vi "mbtestmain.vi"() -> ()   [LabVIEW 2013, in "Modbus Slave tests.lvlib"]
doc: "Platypus Framework 1.0.1.65\nNI Systems Engineering - National Instruments"
uses:
  Modbus Slave tests.lvlib
  <vilib>/NI/Module Execution Interface/Engine Runtime/Engine Runtime Interface.lvclass
  <vilib>/NI/Module Execution Interface/Engine Runtime/Execution States.ctl
  execution/Modbus Slave runtime.lvclass
  <vilib>/NI/TBM Engines/Standard Engine/Runtime/Standard Engine Runtime.lvclass
  <vilib>/NI/TBM Modules/CVT Access/module/execution/CVT runtime.lvclass
  <vilib>/NI/Current Value Table/Current Value Table.lvlib
  <vilib>/NI/Current Value Table/DataTypes/Double_Read.vi
  <vilib>/NI/Current Value Table/DataTypes/Double_Write.vi
  <vilib>/NI/Current Value Table/DataTypes/Boolean_Read.vi
  <vilib>/NI/Current Value Table/DataTypes/Boolean_Write.vi
panel:
  in  "D":bool
  out "C":bool
  in  "B":dbl
  out "A":dbl
  in  "stop 2":bool
  out "final error":errorcluster
  in  "stop":bool
  out "runtime error":errorcluster
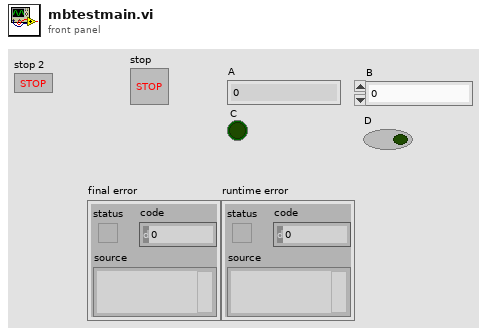
[diagram p1: front panel]
types:
  T1 = typedef "PLConfigurationSerializer.lvlib/systems cluster.ctl" = cluster{"System Configuration":refnum<class "PL_System Configuration.lvclass">, "targets":T2[]}
  T2 = typedef "PLConfigurationSerializer.lvlib/targets cluster.ctl" = cluster{"Target Configuration":refnum<class "PL_Target Configuration.lvclass">, "engines":T3[]}
  T3 = typedef "PLConfigurationSerializer.lvlib/engines cluster.ctl" = cluster{"engine configuration":refnum<class "engine configuration.lvclass">, "modules":refnum<class "TBM module configuration.lvclass">[]}
  T4 = typedef "Engine Runtime Interface.lvclass/Execution States.ctl" = enum16{"Initializing", "Paused (Initialized)", "Running", "Set Safe Outputs", "Uninitializing", "Stopped (Uninitialized)", "Error (Uninitialized)", "Safe State (Uninitialized)", "Closed"}
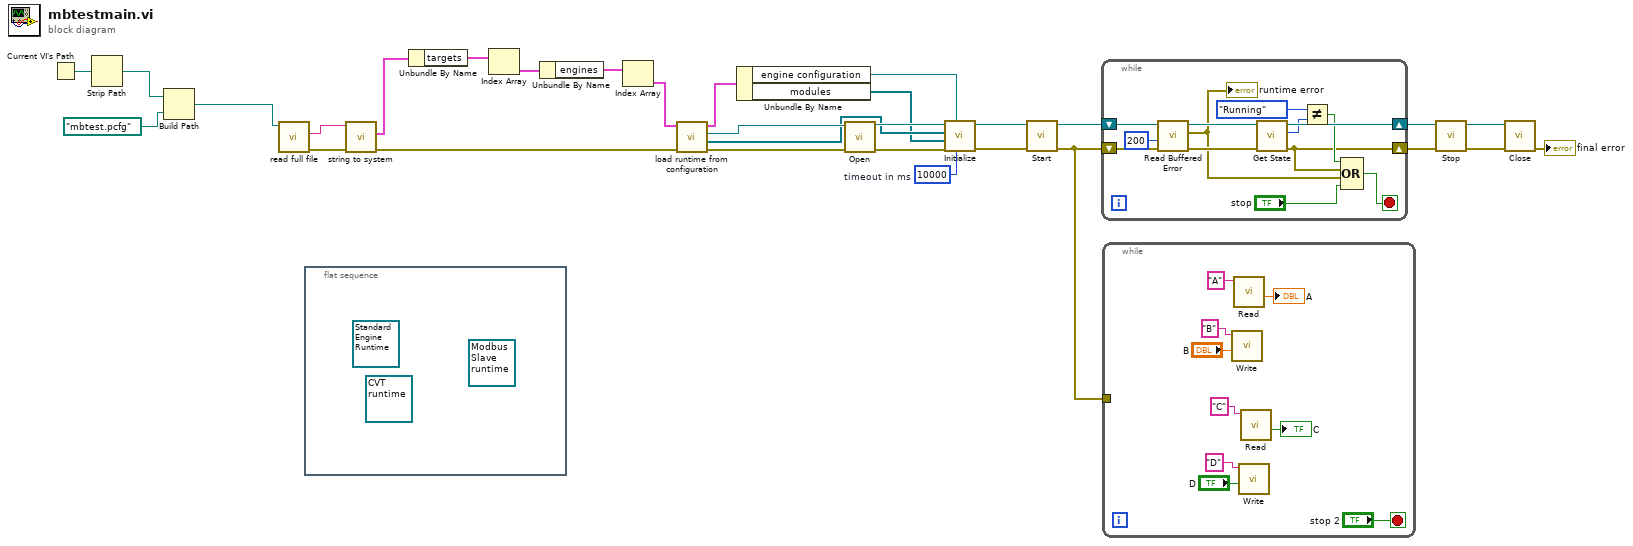
[diagram p0: block diagram]
diagram:
  w16 = 10000  # timeout in ms
  n1 = Current VI's Path() -> (path=w3:path)
  n2 = Strip Path(path=w3) -> (stripped path=w1:path)  [unwired: 1 out]
  n3 = Build Path(base path=w1, name or relative path=path "mbtest.pcfg" ("file path")) -> (appended path=w2:path)
  n4 = call <vilib>:"read full file.vi"("file path"=w2) -> ("error out"=w30:errorcluster, "data"=w29:string)  [unwired: 9 in]
  n5 = flat-sequence {
    frame #0 {
      (unwired) refnum<class "CVT runtime.lvclass"> refnum ("CVT runtime")
      (unwired) refnum<class "Standard Engine Runtime.lvclass"> refnum ("Standard Engine Runtime.lvclass")
      (unwired) refnum<class "Modbus Slave runtime.lvclass"> refnum ("Modbus Slave runtime")
    }
  }
  n6 = call <vilib>:"string to system.vi"("error in"=w30, "data"=w29) -> ("error out"=w25:errorcluster, "system"=w7:T1)  [unwired: 8 in]
  n7 = Unbundle By Name(w7) -> ("targets"=w28:T2[])
  n8 = Index Array(array=w28) -> (element=w27:T2)  [unwired: 1 in]
  n9 = Unbundle By Name(w27) -> ("engines"=w26:T3[])
  n10 = Index Array(array=w26) -> (element=w6:T3)  [unwired: 1 in]
  n11 = call <vilib>:"load runtime from configuration.vi"("error in"=w25, "engine configuration in"=w6) -> ("error out"=w23:errorcluster, "Component Runtime Objects"=w20:refnum<class "TBM module execution interface.lvclass">[], "Engine Runtime Object"=w24:refnum<class "Engine Runtime Interface.lvclass">, "engine configuration out"=w19:T3)  [unwired: 6 in]
  n12 = Unbundle By Name(w19) -> ("engine configuration"=w18:refnum<class "engine configuration.lvclass">, "modules"=w17:refnum<class "TBM module configuration.lvclass">[])
  n13 = call-dynamic "Open.vi"("error in"=w23, "Engine Runtime Interface in"=w24) -> ("error out"=w21:errorcluster, "Engine Runtime Interface out"=w22:refnum<class "Engine Runtime Interface.lvclass">)  [unwired: 8 in]
  n14 = call-dynamic "Initialize.vi"("timeout in ms"=w16, "Engine Configuration"=w18, "error in"=w21, "module Configurations"=w17, "modules"=w20, "Engine Runtime Interface in"=w22) -> ("error out"=w12:errorcluster, "Engine Runtime Interface out"=w13:refnum<class "Engine Runtime Interface.lvclass">)  [unwired: 4 in]
  n15 = call-dynamic "Start.vi"("error in"=w12, "Engine Runtime Interface in"=w13) -> ("error out"=w5:errorcluster, "Engine Runtime Interface out"=w11:refnum<class "Engine Runtime Interface.lvclass">)  [unwired: 8 in]
  n16 = while {
    shift-right: [w39] -> w10
    shift-left: w11 -> [w43]
    shift-right: [w32] -> w9
    shift-left: w5 -> [w42]
    stop <- w37 stop-if-true
    n17 = call-dynamic "Read Buffered Error.vi"("error in"=w42, "timeout in ms (0)"=200, "Engine Runtime Interface in"=w43) -> ("error out"=w40:errorcluster, "Engine Error"=w36:errorcluster, "Engine Runtime Interface out"=w41:refnum<class "Engine Runtime Interface.lvclass">)  [unwired: 6 in]
    "runtime error" <- w36
    n18 = call-dynamic "Get State.vi"("error in"=w40, "Engine Runtime Interface in"=w41) -> ("error out"=w32:errorcluster, "Engine State"=w35:T4, "Engine Runtime Interface out"=w39:refnum<class "Engine Runtime Interface.lvclass">)  [unwired: 7 in]
    n19 = Not Equal?(x=Execution_States."Running" ("Engine State"), y=w35) -> (x != y?=w33:bool)
    n20 = Compound Arithmetic op=OR(w33, w32, w36, "stop") -> (w37:bool)
  }
  n21 = while {
    tunnel: w5 -> [_]
    stop <- "stop 2" stop-if-true
    n22 = call-poly <vilib>:"Write.vi"("Value"="B", "Tag Name"="B") -> ()  [unwired: 9 in, 1 out]
    n23 = call-poly <vilib>:"Read.vi"("Tag Name"="A") -> ("Value"=→"A":dbl)  [unwired: 9 in, 1 out]
    n24 = call-poly <vilib>:"Write.vi"("Value"="D", "Tag Name"="D") -> ()  [unwired: 9 in, 1 out]
    n25 = call-poly <vilib>:"Read.vi"("Tag Name"="C") -> ("Value"=→"C":bool)  [unwired: 9 in, 1 out]
  }
  n26 = call-dynamic "Stop.vi"("error in"=w9, "Engine Runtime Interface in"=w10) -> ("error out"=w14:errorcluster, "Engine Runtime Interface out"=w15:refnum<class "Engine Runtime Interface.lvclass">)  [unwired: 8 in]
  n27 = call-dynamic "Close.vi"("error in"=w14, "Engine Runtime Interface in"=w15) -> ("error out"=→"final error":errorcluster)  [unwired: 9 in]
